vi "FG - DAQ Error Cluster.vi"(7 "action (Get)":T1=enum."Get", 10 "error":errorcluster) -> (2 "error out":errorcluster)   [LabVIEW 2019, in "DAQ_Engine.lvclass"]
doc: "Developed by Kevin Thompson\nkevin@thompsonengineering.net\n\nCopyright 2020\nThompson Engineering, LLC"
uses:
  DAQ_Engine.lvclass
  Common/DataTypes/TD GetSet ActionSelect--enum.ctl
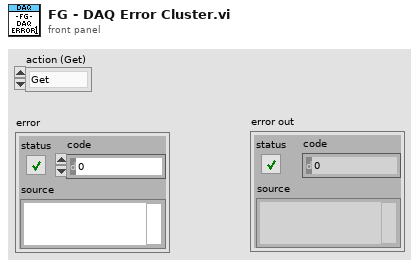
[diagram p1: front panel]
types:
  T1 = typedef "TD GetSet ActionSelect--enum.ctl" = enum16{"Init", "Get", "Set"}
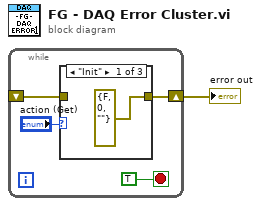
[diagram p0: block diagram]
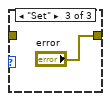
[diagram p3: hidden frame]
diagram:
  n1 = while {
    shift-right: [w3] -> w1
    shift-left: _ -> [w2]
    stop <- TRUE stop-if-true
    n2 = case shown="\"Init\"" "action (Get)" {
      tunnel: [errorcluster {"status"=FALSE, "code"=0, "source"=""} ("error constant") w7 "error"] -> w3
      tunnel: w2 -> [_ w7 _]
      frame "Init" {
      }
      frame "Get", Default {
      }
      frame "Set" {
      }
    }
  }
  "error out" <- w1
